vi "SDG Check Physical Channel Port.vi"(0 "Physical Channel In":tag, 11 "error in (no error)":errorcluster) -> (4 "Physical Channel Out":tag, 15 "error out":errorcluster)   [LabVIEW 2021, in "DAQ_Static Digital State Generation.lvlib"]
doc: "Checks for the presence of port in the physical channel input and throws the required error when identified."
uses:
  DAQ_Static Digital State Generation.lvlib
  <vilib>/Utility/error.llb/Error Cluster From Error Code.vi
  <vilib>/ErrorRing/Error Ring.xnode
  <resource>/objmgr/daqmx.rc
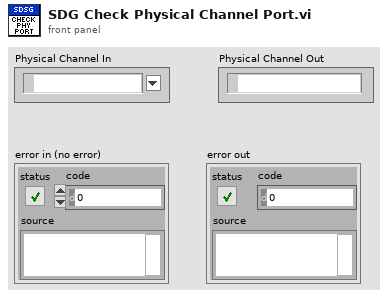
[diagram p1: front panel]
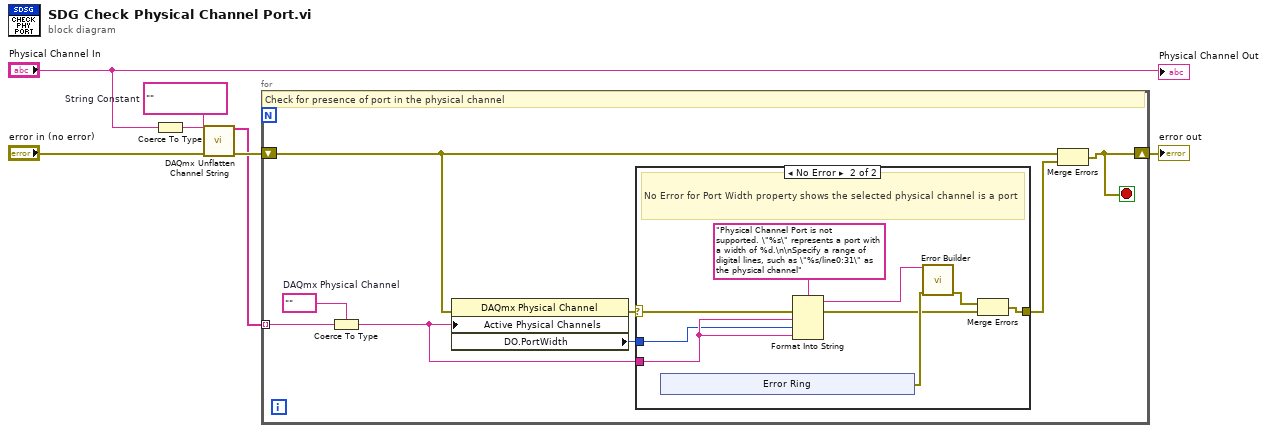
[diagram p0: block diagram]
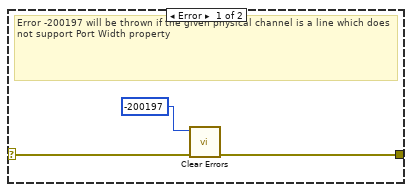
[diagram p2: hidden frame]
diagram:
  w4 = ""  # String Constant
  n1 = Coerce To Type(0:"Physical Channel In", 1:w4) -> (2:w2:string)
  n2 = call <vilib>:"DAQmx Unflatten Channel String.vi"("names in"=w2, "error in"="error in (no error)") -> ("names out"=w6:string[], "error out"=w7:errorcluster)  [unwired: 12 in]
  n3 = for {
    tunnel: w6 -> [w15] mode=indexing
    shift-right: [w11] -> w5
    shift-left: w7 -> [w13]
    stop <- w11 stop-if-true
    w14 = tag ""  # DAQmx Physical Channel
    # "Check for presence of port in the physical channel"
    n4 = Coerce To Type(0:w15, 1:w14) -> (2:w8:tag)
    n5 = property class="DAQmx Physical Channel"(error in=w13, "Active Physical Channels"=w8) -> (error out=w9:errorcluster, "DO.PortWidth"=w10:u32)  [unwired: 1 in, 1 out]
    n6 = case shown="No Error" w9 {
      selector: w9 -> [w18 w22]
      tunnel: [w17 w19] -> w12
      tunnel: w10 -> [_ w20]
      tunnel: w8 -> [_ w21]
      frame Error {
        # "Error -200197 will be thrown if the given physical channel is a line which does not support Port Width property"
        n7 = call <vilib>:"Clear Errors.vi"("error in (no error)"=w18, "specific error code to clear (0: all)"=-200197) -> ("error out"=w17:errorcluster)  [unwired: 4 in, 1 out]
      }
      frame No Error {
        # "No Error for Port Width property shows the selected physical channel is a port"
        n8 = xnode "Error Ring"() -> ("error out"=w25:errorcluster)
        n9 = Format Into String(format string="Physical Channel Port is not supported. \"%s\" represents a port with a width of %d.\n\nSpecify a range of digital lines, such as \"%s/line0:31\" as the physical channel" ("error message (\"\")"), error in=w22, w21, w20, w21) -> (resulting string=w26:string, error out=w23:errorcluster)  [unwired: 1 in]
        n10 = call "Error Builder.vi"("Error String"=w26, "Error In"=w25) -> ("Error Out"=w24:errorcluster)  [unwired: 13 in]
        n11 = Merge Errors(w24, w23) -> (w19:errorcluster)
      }
    }
    n12 = Merge Errors(w13, w12) -> (w11:errorcluster)
  }
  "error out" <- w5
  "Physical Channel Out" <- "Physical Channel In"
